vi "change_decorations_colors.vi"() -> ()   [LabVIEW 2011]
doc: "This VI shows how to change the color of a decoration. Knowing how to change the color, any other property can be also change.\n1. Select FIRST the Color\n2. Run VI"
panel:
  in  "Decorations Color":u32(colorbox)
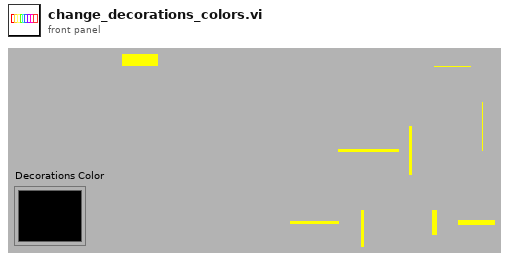
[diagram p1: front panel]
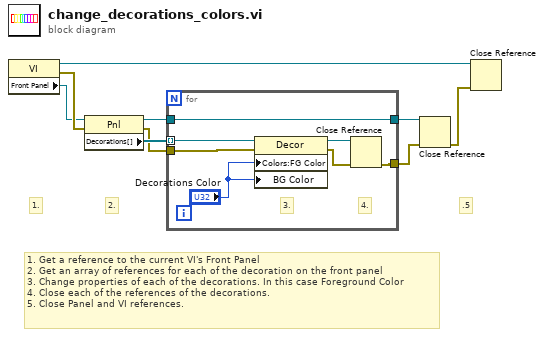
[diagram p0: block diagram]
diagram:
  # "1. Get a reference to the current VI's Front Panel\n2. Get an array of references for each of the decoration on the front panel\n3. Change properties of each of the decorations. In this case Foreground Color\n4. Close each of the references of the decorations.\n5. Close Panel and VI references."
  # ".5"
  # "2."
  # "1."
  n1 = property class="VI"() -> (reference out=w1:refnum<vi>, error out=w9:errorcluster, "Front Panel"=w8:refnum<vi>)  [unwired: 2 in]
  n2 = property class="Pnl"(reference=w8, error in=w9) -> (reference out=w5:refnum<vi>, error out=w6:errorcluster, "Decorations[]"=w7:refnum<vi>[])
  n3 = for {
    tunnel: w7 -> [w16] mode=indexing
    tunnel: w6 -> [w13]
    tunnel: w5 -> [w12]
    tunnel: [w12] -> w4
    tunnel: [w11] -> w3
    # "4."
    # "3."
    n4 = property class="Decor"(reference=w16, error in=w13, "Colors:FG Color"="Decorations Color", "BG Color"="Decorations Color") -> (reference out=w15:refnum<vi>, error out=w14:errorcluster)
    n5 = Close Reference(reference=w15, error in (no error)=w14) -> (error out=w11:errorcluster)
  }
  n6 = Close Reference(reference=w4, error in (no error)=w3) -> (error out=w2:errorcluster)
  n7 = Close Reference(reference=w1, error in (no error)=w2) -> ()  [unwired: 1 out]
